vi "DetectPressureAnomalies.vi"(3 "Pressure Loss Threshold (psi/min)":dbl=-5.0, 4 "Compressor Running":bool, 5 "Pressure (psi)":dbl(slide) scale=0.0..120.0) -> (0 "Pressure Change (psi/min)":dbl, 1 "Pressure Leak":bool, 2 "Pressure Vent":bool)   [LabVIEW 2019]
doc: "This VI can detect both rapid pressure venting events and slow pressure leak conditions."
uses:
  <vilib>/Analysis/NI_AALPro.lvlib
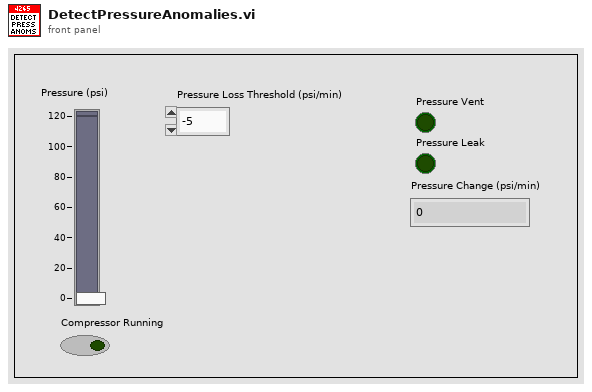
[diagram p1: front panel]
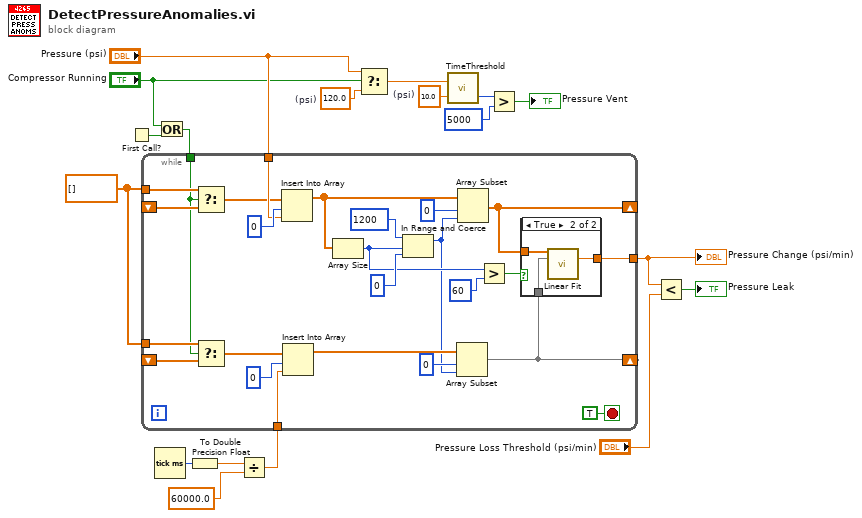
[diagram p0: block diagram]
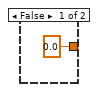
[diagram p2: hidden frame]
diagram:
  w4 = dbl[] [] ("array")
  w17 = 120.0  # (psi)
  w18 = 10.0  # (psi)
  n1 = First Call?() -> (First Call?: T/F=w11:bool)
  n2 = Tick Count (ms)() -> (millisecond timer value=w8:u32)
  n3 = Or(x="Compressor Running", y=w11) -> (x .or. y?=w9:bool)
  n4 = To Double Precision Float(number=w8) -> (double precision float=w7:dbl)
  n5 = Divide(x=w7, y=60000.0) -> (x/y=w5:dbl)
  n6 = while {
    tunnel: "Pressure (psi)" -> [w41]
    shift-right: [w34] -> _
    shift-left: _ -> [w40]
    tunnel: w4 -> [w39]
    tunnel: w9 -> [w22]
    tunnel: [w30] -> w3
    tunnel: w5 -> [w27]
    tunnel: w4 -> [w24]
    shift-right: [w20] -> _
    shift-left: _ -> [w19]
    stop <- TRUE stop-if-true
    n7 = Select(t=w39, s=w22, f=w40) -> (s? t:f=w28:dbl[])
    n8 = Select(t=w24, s=w22, f=w19) -> (s? t:f=w23:dbl[])
    n9 = Insert Into Array(array=w28, index=0, new element=w41) -> (w37:dbl[])
    n10 = Insert Into Array(array=w23, index=0, new element=w27) -> (w25:dbl[])
    n11 = Array Size(array=w37) -> (size(s)=w32:i32)
    n12 = In Range and Coerce(upper limit=1200, x=w32, lower limit=0) -> (coerced(x)=w21:i32)  [unwired: 1 out]
    n13 = Array Subset(array=w25, index=0, length=w21) -> (w20:dbl[])
    n14 = Array Subset(array=w37, index=0, length=w21) -> (w34:dbl[])
    n15 = Greater?(x=w32, y=60) -> (0:w33:bool)
    n16 = case shown="True" w33 {
      tunnel: w34 -> [_ w47]
      tunnel: [0.0 ("slope") w46] -> w30
      tunnel: w20 -> [_ w45]
      frame False {
      }
      frame True {
        n17 = call <vilib>:"Linear Fit.vi"("Y"=w47, "X"=w45) -> ("slope"=w46:dbl)  [unwired: 9 in, 4 out]
      }
    }
  }
  "Pressure Change (psi/min)" <- w3
  n18 = Select(t="Pressure (psi)", s="Compressor Running", f=w17) -> (s? t:f=w16:dbl)
  n19 = call "TimeThreshold.vi"("Threshold"=w18, "Current Value"=w16) -> ("Time Below Threshold (ms)"=w15:u32)  [unwired: 1 out]
  n20 = Greater?(x=w15, y=u32 5000) -> (0:→"Pressure Vent":bool)
  n21 = Less?(x=w3, y="Pressure Loss Threshold (psi/min)") -> (x < y?=→"Pressure Leak":bool)
